vi "LV FPGA Serial Read-James'.vi"(1 "Read FIFO":refnum<k21>="Read FIFO", 5 "Receive":refnum<k21>="Port8/DIOCTL", 7 "baud rate (9600)":u32=9600, 9 "data bits (8)":i32=8 min=5 max=8 step=1, 11 "parity (0:none)":enum16{"None", "Odd", "Even", "Mark", "Space"}(ring), 12 "stop bits (10: 1 bit)":u16(ring)=10 items=["1.0"=10, "1.5"=15, "2.0"=20], 13 "Invert Polarity?":bool) -> ()   [LabVIEW 2010]
uses:
  <vilib>/eio/EIONode/EIONode.xnode
  <vilib>/rvi/eio/nirviEIOImplementation/nirviEIOImplementation.xnode
  <vilib>/rvi/eio/common/nirviEmuClasses.ctl
  <vilib>/rvi/DataTransferAndStorage/Container/XNode/niFpgaContainer.xnode
  <vilib>/rvi/DataTransferAndStorage/Container/Common/niFpgaTransferTypeControl.ctl
  <vilib>/rvi/FIFO/Fifo_Types/niFpgaFifoControlLogicControl.ctl
  <vilib>/rvi/DataTransferAndStorage/Container/Common/niFpgaContainerMethod.ctl
  <vilib>/rvi/DataTransferAndStorage/Container/Common/niFpgaContainerMetaDataKey.ctl
  <vilib>/rvi/DataTransferAndStorage/FIFO/niFpgaPeerToPeerStreamState.ctl
  1.0-Hindbrain Global.vi
  <vilib>/rvi/eio/common/nirviEmuTemplateMethod_noerrors.vi
  Instance           1 27Saved   LV FPGA Serial Read .vi
  Instance           2 27Saved   LV FPGA Serial Read .vi
  <vilib>/rvi/DataTransferAndStorage/Container/Common/niFpgaContainerExecOnDevCompGetState.vi
  <vilib>/rvi/FIFO/Fifo_Resource/nirvififoEmulationSetSize.vi
  <vilib>/rvi/DataTransferAndStorage/Container/Common/niFpgaContainerGetUniqueNameForEmu.vi
  <vilib>/rvi/interface/RandomDataEmulation/nirviRandomDataFPGAFIFO.vi
  <vilib>/rvi/interface/RandomDataEmulation/niFpgaRandomDataHandleErrors.vi
  <vilib>/rvi/eio/common/nirviEmuReportErrorAndStop.vi
  Instance           3 27Saved   LV FPGA Serial Read .vi
  Instance           6 27Saved   LV FPGA Serial Read .vi
panel:
  out "Read: Transmission Error":bool
  in  "stop":bool
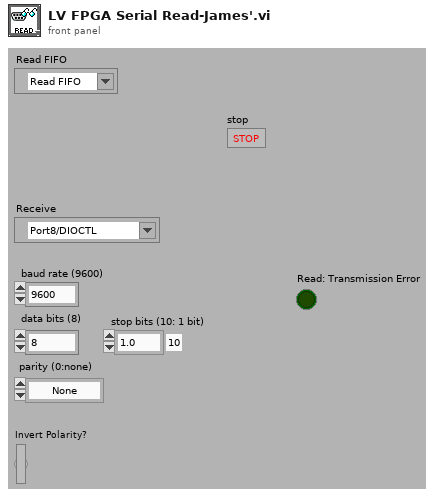
[diagram p1: front panel]
types:
  T1 = typedef "nirviEmuClasses.ctl" = enum16{"IO Read", "IO Write", "Method", "Property Read", "Property Write"}
  T2 = typedef "niFpgaFifoControlLogicControl.ctl" = enum16{"Slice Fabric", "Target Optimal", "Built-in"}
  T3 = typedef "niFpgaContainerMethod.ctl" = enum16{"<none>", "write", "read", "clear", "getNumberOfElementsToWrite", "getNumberOfElementsToRead", "enable", "disable", "flushAndDisable", "getStreamState", "readA", "readB", "dramWrite", "dramWriteWithByteEnables", "dramRequestData", "dramRetrieveData"}
  T4 = typedef "niFpgaTransferTypeControl.ctl" = enum16{"Target-Scoped", "Host to Target - DMA", "Target to Host - DMA", "Peer to Peer Reader", "Peer to Peer Writer", "Bidirectional"}
  T5 = typedef "niFpgaPeerToPeerStreamState.ctl" = enum16{"Unlinked", "Disabled", "Enabled", "Flushing"}
  T6 = typedef "niFpgaContainerMetaDataKey.ctl" = enum16{"FPGA FIFO", "FPGA Memory", "FPGA Register"}
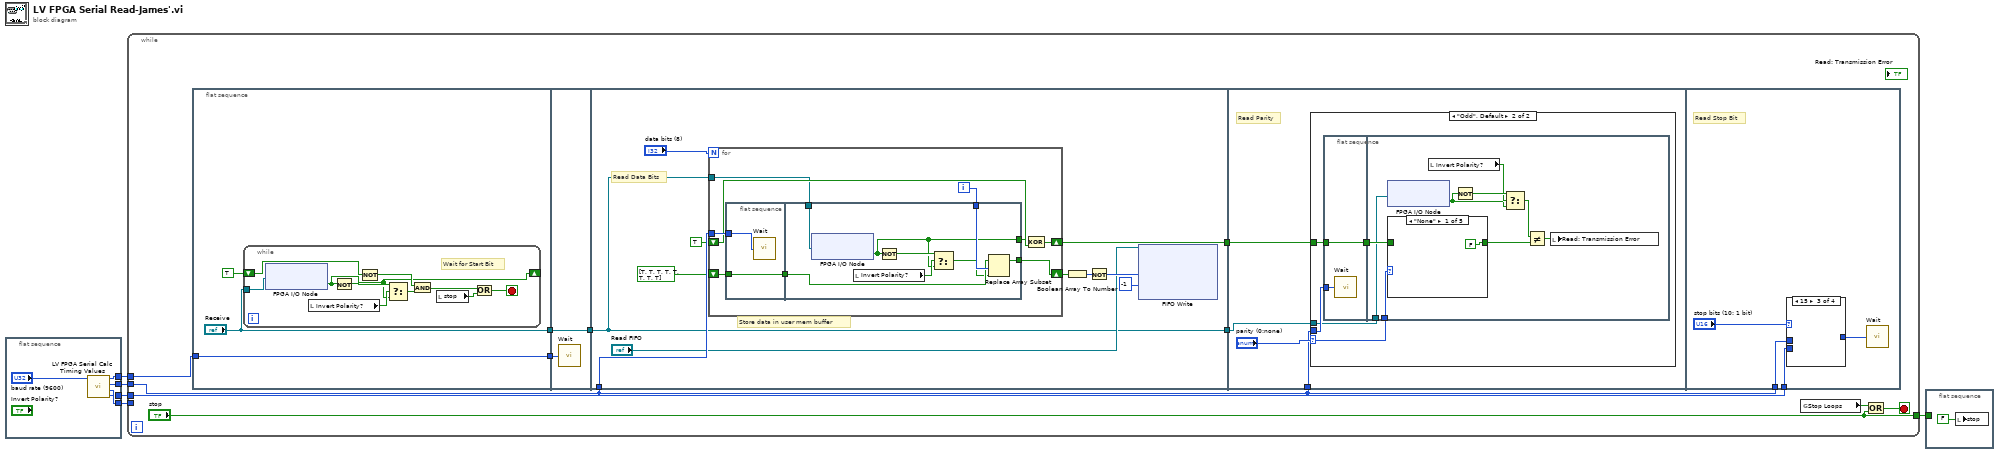
[diagram p0: block diagram]
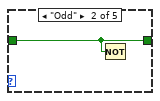
[diagram p3: hidden frame]
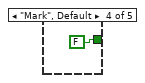
[diagram p5: hidden frame]
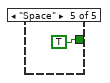
[diagram p6: hidden frame]
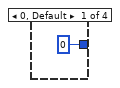
[diagram p7: hidden frame]
diagram:
  n1 = flat-sequence {
    tunnel: [w6] -> w4
    tunnel: [w9] -> w5
    tunnel: [w8] -> w3
    tunnel: [w7] -> w2
    frame #0 {
      n2 = call "LV FPGA Serial Calc Timing Values.vi"("baud rate (1000000)"="baud rate (9600)") -> ("Two Bit"=w7:u32, "One and Half Bit"=w8:u32, "One Bit"=w6:u32, "Half Bit"=w9:u32)  [unwired: 1 in, 2 out]
    }
  }
  n3 = while {
    tunnel: w2 -> [w21]
    tunnel: w3 -> [_]
    tunnel: w4 -> [w20]
    tunnel: w5 -> [w19]
    tunnel: ["stop"] -> w1
    stop <- w16 stop-if-true
    n4 = flat-sequence {
      tunnel: w19 -> [w24]
      tunnel: [w24] -> w14
      tunnel: ["Receive"] -> w12
      tunnel: w14 -> [w57]
      tunnel: [w56] -> w13
      tunnel: w12 -> [w56]
      tunnel: w20 -> [w68]
      tunnel: [w64] -> w15
      tunnel: w13 -> [w59]
      tunnel: [w59] -> w11
      tunnel: w20 -> [w427]
      tunnel: w15 -> [w429]
      tunnel: w11 -> [w426]
      tunnel: w20 -> [w474]
      tunnel: w21 -> [w473]
      frame #0 {
        n5 = while {
          shift-right: [w25] -> _
          shift-left: TRUE -> [w34]
          tunnel: "Receive" -> [w29]
          stop <- w30 stop-if-true
          # "Wait for Start Bit"
          n6 = xnode "FPGA I/O Node"("FPGA I/O In"=w29) -> ("I/O Item"=w25:bool)  [unwired: 1 out]
          n7 = local read "Invert Polarity?"() -> (w27:bool)
          n8 = Not(x=w25) -> (.not. x?=w28:bool)
          n9 = Not(x=w34) -> (.not. x?=w33:bool)
          n10 = Select(t=w28, s=w27, f=w25) -> (s? t:f=w26:bool)
          n11 = And(x=w33, y=w26) -> (x .and. y?=w31:bool)
          n12 = local read "stop"() -> (w32:bool)
          n13 = Or(x=w31, y=w32) -> (x .or. y?=w30:bool)
        }
      }
      frame #1 {
        n14 = call "Wait"("Count(Ticks)"=w57) -> ()  [unwired: 1 out]
      }
      frame #2 {
        # "Store data in user mem buffer"
        # "Read Data Bits"
        n15 = for {
          N: "data bits (8)" -> [_]
          shift-right: [w388] -> w67
          shift-left: bool[] [TRUE, TRUE, TRUE, TRUE, TRUE, TRUE, TRUE, TRUE] -> [w394]
          tunnel: w68 -> [w392]
          shift-right: [w391] -> w64
          shift-left: TRUE -> [w390]
          tunnel: w59 -> [w386]
          i -> [w387]
          n16 = flat-sequence {
            tunnel: w394 -> [w396]
            tunnel: [w396] -> w393
            tunnel: w392 -> [w395]
            tunnel: w387 -> [w404]
            tunnel: w393 -> [w403]
            tunnel: [w402] -> w388
            tunnel: [w397] -> w389
            tunnel: w386 -> [w401]
            frame #0 {
              n17 = call "Wait"("Count(Ticks)"=w395) -> ()  [unwired: 1 out]
            }
            frame #1 {
              n18 = xnode "FPGA I/O Node"("FPGA I/O In"=w401) -> ("I/O Item"=w397:bool)  [unwired: 1 out]
              n19 = local read "Invert Polarity?"() -> (w400:bool)
              n20 = Not(x=w397) -> (.not. x?=w399:bool)
              n21 = Select(t=w399, s=w400, f=w397) -> (s? t:f=w398:bool)
              n22 = Replace Array Subset(array=w403, new element=w398, index=w404) -> (w402:bool[])
            }
          }
          n23 = Exclusive Or(1:w390, 2:w389) -> (0:w391:bool)
        }
        n24 = Boolean Array To Number(Boolean array=w67) -> (number=w66:u8)
        n25 = Not(x=w66) -> (.not. x?=w62:u8)
        n26 = xnode ("FIFO Write")("Element"=w62, "Timeout"=-1, "FIFO In"="Read FIFO") -> ()  [unwired: 2 out]
      }
      frame #3 {
        # "Read Parity"
        n27 = case shown="\"Odd\", Default" "parity (0:none)" {
          selector: "parity (0:none)" -> [_ w433]
          tunnel: w429 -> [_ w431]
          tunnel: w427 -> [_ w434]
          tunnel: w426 -> [_ w430]
          frame "None" {
          }
          frame "Odd", Default {
            n28 = flat-sequence {
              tunnel: w434 -> [w436]
              tunnel: [w435] -> w432
              tunnel: w431 -> [w435]
              tunnel: w433 -> [w445]
              tunnel: w432 -> [w443]
              tunnel: w430 -> [w441]
              frame #0 {
                n29 = call "Wait"("Count(Ticks)"=w436) -> ()  [unwired: 1 out]
              }
              frame #1 {
                n30 = xnode "FPGA I/O Node"("FPGA I/O In"=w441) -> ("I/O Item"=w438:bool)  [unwired: 1 out]
                n31 = case shown="\"None\"" w445 {
                  tunnel: w443 -> [_ w468 w469 _ _]
                  tunnel: [FALSE ("y") w468 w469 FALSE ("y") TRUE ("y")] -> w444
                  frame "None" {
                  }
                  frame "Odd" {
                    n32 = Not(x=w468) -> ()  [unwired: 1 out]
                  }
                  frame "Even" {
                  }
                  frame "Mark", Default {
                  }
                  frame "Space" {
                  }
                }
                n33 = local read "Invert Polarity?"() -> (w439:bool)
                n34 = Not(x=w438) -> (.not. x?=w440:bool)
                n35 = Select(t=w440, s=w439, f=w438) -> (s? t:f=w437:bool)
                n36 = Not Equal?(x=w437, y=w444) -> (x != y?=w442:bool)
                n37 = local write "Read: Transmission Error"(w442) -> ()
              }
            }
          }
        }
      }
      frame #4 {
        # "Read Stop Bit"
        n38 = case shown="15" "stop bits (10: 1 bit)" {
          tunnel: w474 -> [_ w477 _ _]
          tunnel: w473 -> [_ _ _ w478]
          tunnel: [u32 0 ("One Bit") w477 _ w478] -> w472
          frame 0, Default {
          }
          frame 10 {
          }
          frame 15 {
          }
          frame 20 {
          }
        }
        n39 = call "Wait"("Count(Ticks)"=w472) -> ()  [unwired: 1 out]
      }
    }
    n40 = global read "1.0-Hindbrain Global.vi" "Stop Loops"() -> (w18:bool)
    n41 = Or(x=w18, y="stop") -> (x .or. y?=w16:bool)
  }
  n42 = flat-sequence {
    tunnel: w1 -> [_]
    frame #0 {
      n43 = local write "stop"(FALSE ("stop")) -> ()
    }
  }
